vi "DSF.Memory.Buffer.Config.Get Channel Count.vi"(8 "error in (no error)":errorcluster, 11 "Buffer Config in":refnum<class "DSF.Memory.Buffer.Config.lvclass">) -> (0 "error out":errorcluster, 2 "channel count":u64 format="%d channels", 3 "Buffer Config out":refnum<class "DSF.Memory.Buffer.Config.lvclass">)   [LabVIEW 2016, in "DSF.Memory.lvlib" / "DSF.Memory.Buffer.Config.lvclass"]
uses:
  DSF.Memory.Buffer.Config.lvclass
  DSF.Memory.Buffer.Config.lvclass/DSF.Memory.Buffer.Config.ctl
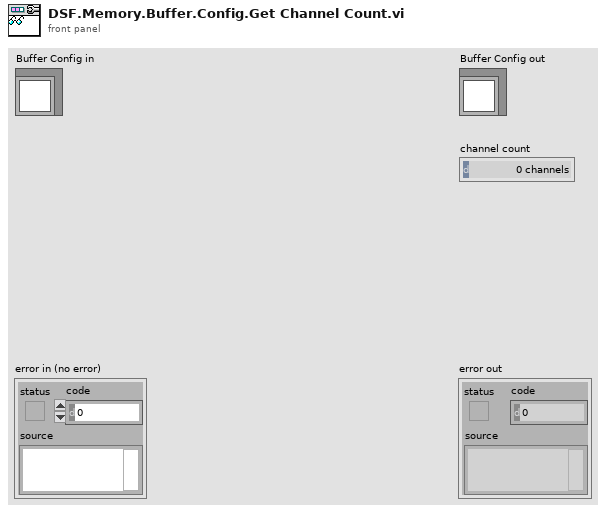
[diagram p1: front panel]
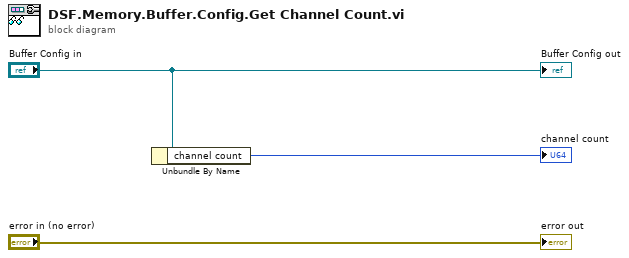
[diagram p0: block diagram]
diagram:
  n1 = Unbundle By Name("Buffer Config in") -> ("channel count"=→"channel count":u64)
  "error out" <- "error in (no error)"
  "Buffer Config out" <- "Buffer Config in"
